vi "Build DashBoard Data.vi"(11 "Dashboard Enables":T2={"Analog Module 1"=[TRUE, TRUE, TRUE, TRUE, TRUE, TRUE, TRUE, TRUE], "Analog Module 2"=[FALSE, FALSE, FALSE, FALSE, FALSE, FALSE, FALSE, FALSE], "Digital Module 1"=TRUE, "Digital Module 2"=FALSE, "Solenoid Module"=TRUE}) -> ()   [LabVIEW 2011]
doc: "This VI builds data and sends it back to the dashboard PC program. By default it sends back the raw values for the first analog, digital, and solenoid module. Modify it to send back the data you want to view. Consider adding higher level data to the Dashboard Datatype.ctl and to this VI. Then update the Dashboard to display the data however you like.\n\nThis software is licensed. Open the labview\\readme\\WPI Robotics Library Open Source License.txt file for more information."
uses:
  DashboardEnable.ctl
  Dashboard Datatype.ctl
  <vilib>/Rock Robotics/WPI/DriverStation/WPI_DriverStationDigitalData.ctl
  System Set Points and States.vi
panel:
  out "Dashboard Data":T1
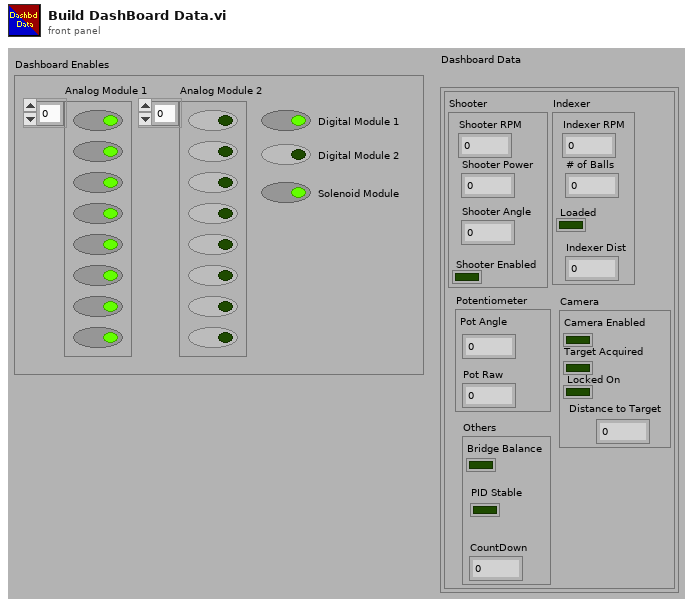
[diagram p1: front panel]
types:
  T1 = typedef "Dashboard Datatype.ctl" = cluster{"Robot Outputs":cluster{"Shooter":cluster{"Shooter RPM":dbl, "Shooter Angle":dbl, "Shooter Power":dbl, "Shooter Enabled":bool}, "Indexer":cluster{"Indexer RPM":dbl, "Loaded":bool, "# of Balls":dbl, "Indexer Dist":dbl}, "Camera":cluster{"Locked On":bool, "Target Acquired":bool, "Camera Enabled":bool, "Distance to Target":dbl}, "Potentiometer":cluster{"Pot Raw":dbl, "Pot Angle":dbl}, "Others":cluster{"CountDown":dbl, "Bridge Balance":bool, "PID Stable":bool}}}
  T2 = typedef "DashboardEnable.ctl" = cluster{"Analog Module 1":bool[], "Analog Module 2":bool[], "Digital Module 1":bool, "Digital Module 2":bool, "Solenoid Module":bool}
  T3 = typedef "WPI_DriverStationDigitalData.ctl" = cluster{"Relay Fwd":u8, "Relay Rev":u8, "GPIO":u16, "GPIO_OE":u16, "PWM":cluster{"PWM[0]":u8, "PWM[1]":u8, "PWM[2]":u8, "PWM[3]":u8, "PWM[4]":u8, "PWM[5]":u8, "PWM[6]":u8, "PWM[7]":u8, "PWM[8]":u8, "PWM[9]":u8}}
  T4 = cluster{"Shooter":cluster{"Shooter RPM":dbl, "Shooter Angle":dbl, "Shooter Power":dbl, "Shooter Enabled":bool}, "Indexer":cluster{"Indexer RPM":dbl, "Loaded":bool, "# of Balls":dbl, "Indexer Dist":dbl}, "Camera":cluster{"Locked On":bool, "Target Acquired":bool, "Camera Enabled":bool, "Distance to Target":dbl}, "Potentiometer":cluster{"Pot Raw":dbl, "Pot Angle":dbl}, "Others":cluster{"CountDown":dbl, "Bridge Balance":bool, "PID Stable":bool}}
  T5 = cluster{"Shooter RPM":dbl, "Shooter Angle":dbl, "Shooter Power":dbl, "Shooter Enabled":bool}
  T6 = cluster{"Indexer RPM":dbl, "Loaded":bool, "# of Balls":dbl, "Indexer Dist":dbl}
  T7 = cluster{"Locked On":bool, "Target Acquired":bool, "Camera Enabled":bool, "Distance to Target":dbl}
  T8 = cluster{"CountDown":dbl, "Bridge Balance":bool, "PID Stable":bool}
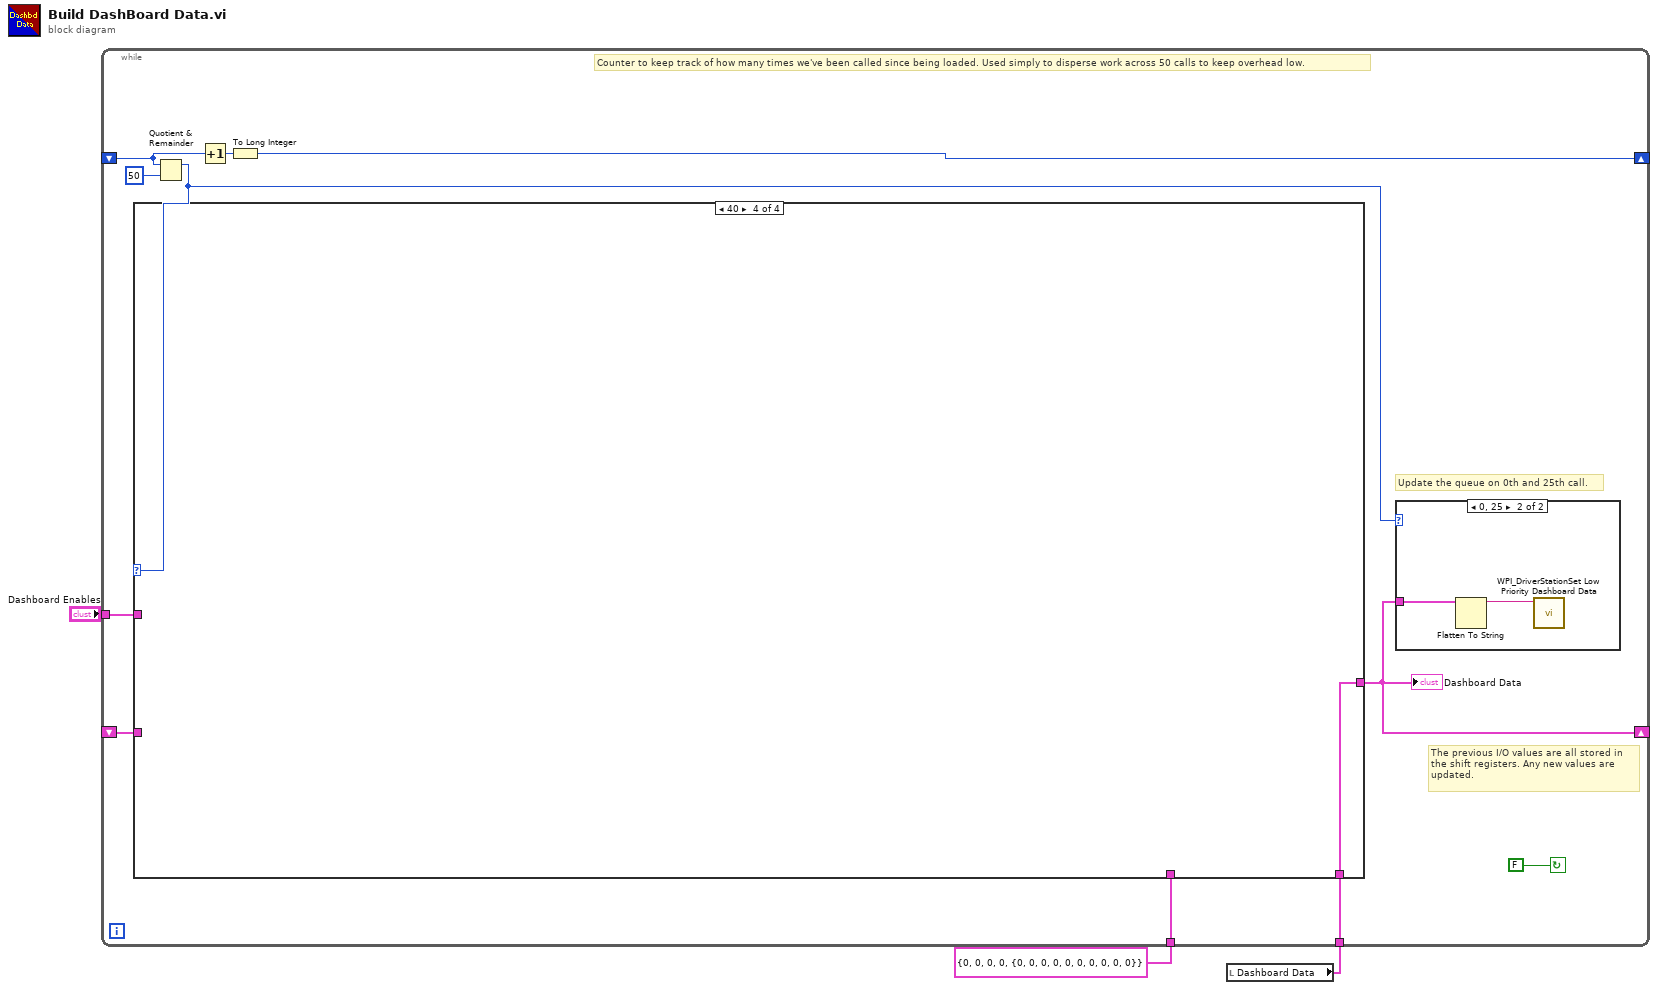
[diagram p0: block diagram]
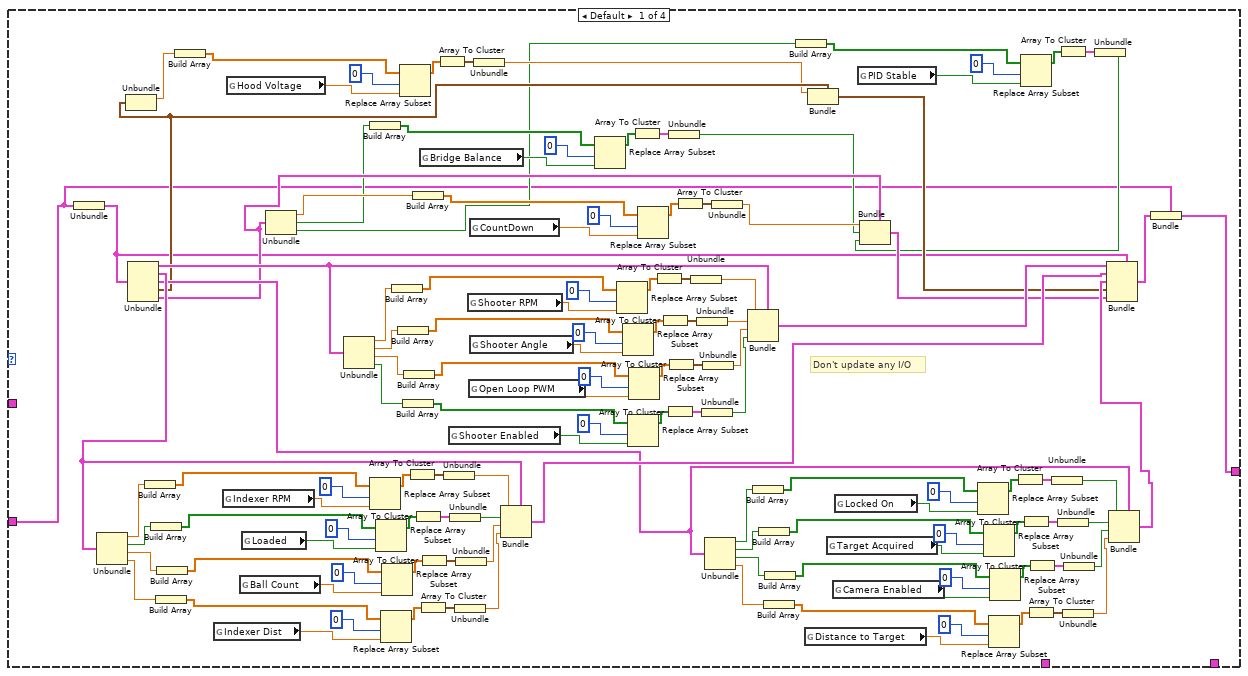
[diagram p3: hidden frame]
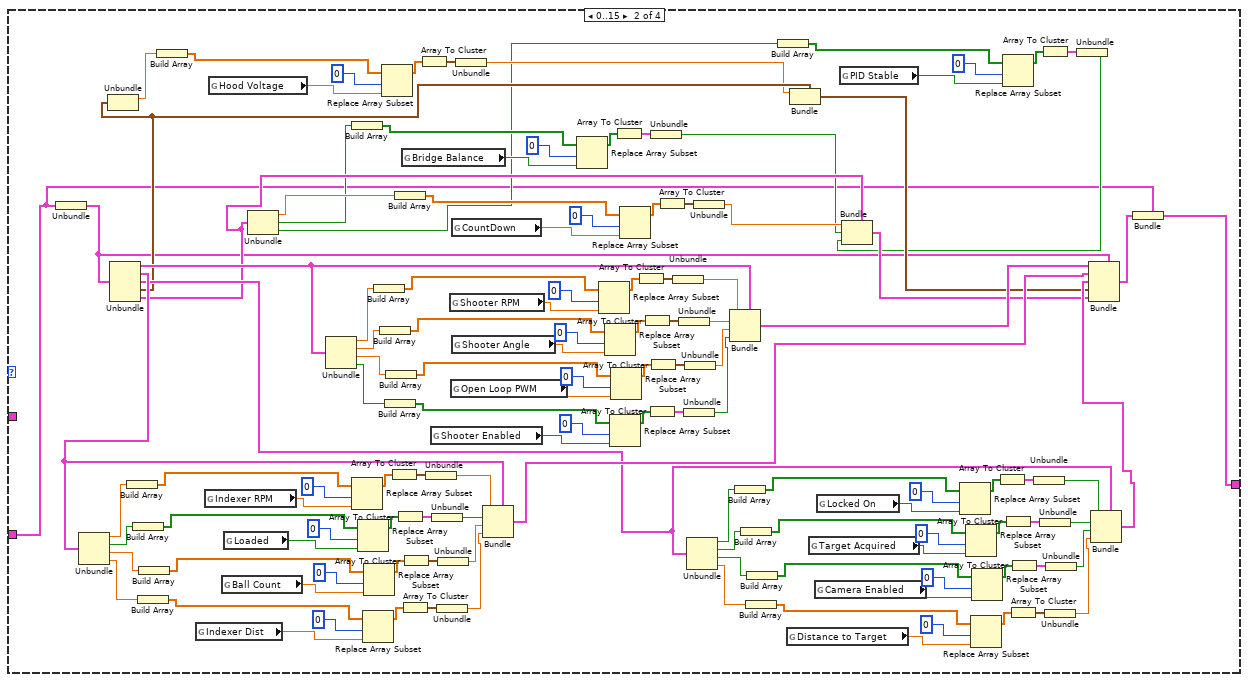
[diagram p4: hidden frame]
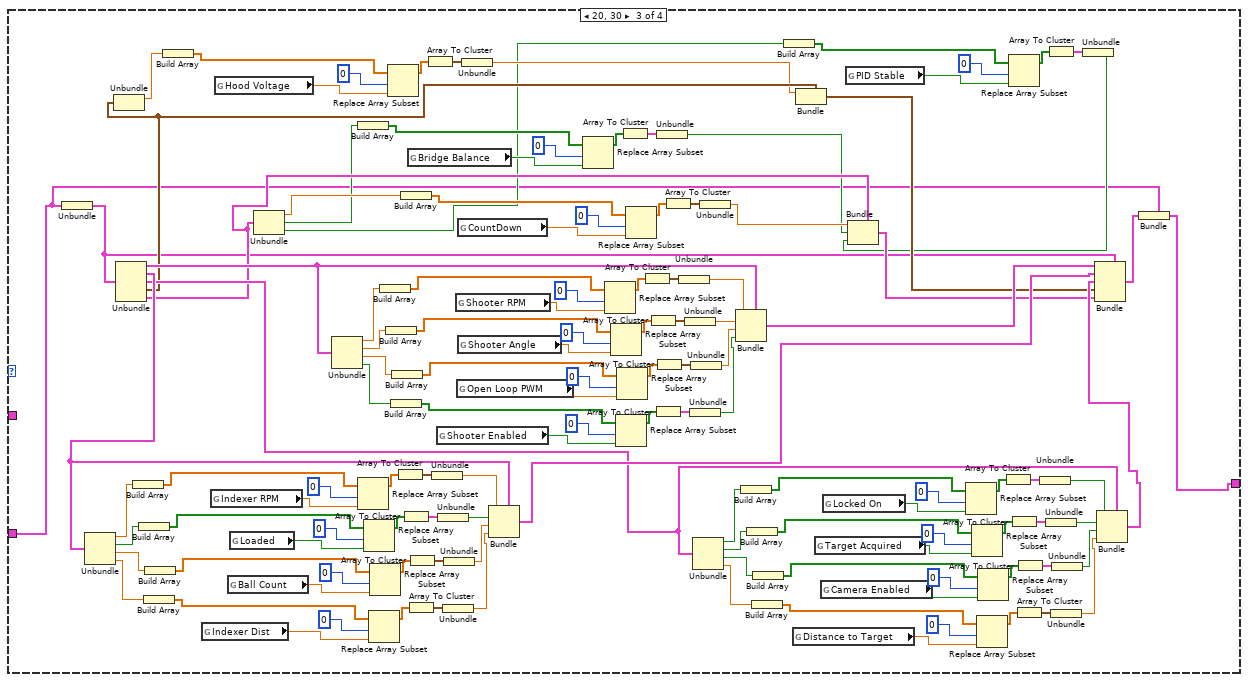
[diagram p5: hidden frame]
diagram:
  n1 = local read "Dashboard Data"() -> (w2:T1)
  n2 = while {
    shift-right: [w7] -> _
    shift-left: _ -> [w9]
    shift-right: [w4] -> _
    shift-left: _ -> [w12]
    tunnel: T3 {"Relay Fwd"=0, "Relay Rev"=0, "GPIO"=0, "GPIO_OE"=0, "PWM"={"PWM[0]"=0, "PWM[1]"=0, "PWM[2]"=0, "PWM[3]"=0, "PWM[4]"=0, "PWM[5]"=0, "PWM[6]"=0, "PWM[7]"=0, "PWM[8]"=0, "PWM[9]"=0}} ("DigitalModule[1]") -> [w11]
    tunnel: w2 -> [w6]
    tunnel: "Dashboard Enables" -> [w5]
    stop <- FALSE continue-if-true
    # "Counter to keep track of how many times we've been called since being loaded. Used simply to disperse work across 50 calls to keep overhead low."
    # "Update the queue on 0th and 25th call."
    # "The previous I/O values are all stored in\nthe shift registers. Any new values are\nupdated."
    n3 = Quotient & Remainder(x=w9, y=50) -> (x-y*floor(x/y)=w8:i32)  [unwired: 1 out]
    n4 = case shown="40" w8 {
      tunnel: [w17 w146 w269 w395] -> w4
      tunnel: w12 -> [w18 w145 w270 _]
      tunnel: w11 -> [_ _ _ _]
      tunnel: w6 -> [_ _ _ w395]
      tunnel: w5 -> [_ _ _ _]
      frame Default {
        # "Don't update any I/O"
        n5 = Unbundle(w18) -> ("Robot Outputs"=w20:T4)
        n6 = Unbundle(w20) -> ("Shooter"=w141:T5, "Indexer"=w84:T6, "Camera"=w54:T7, "Potentiometer"=w31:cluster{"Pot Raw":dbl, "Pot Angle":dbl}, "Others"=w46:T8)
        n7 = Unbundle(w84) -> ("Indexer RPM"=w106:dbl, "Loaded"=w100:bool, "# of Balls"=w92:dbl, "Indexer Dist"=w86:dbl)
        n8 = Unbundle(w31) -> ("Pot Raw"=w32:dbl)  [unwired: 1 out]
        n9 = Build Array(w106) -> (w112:dbl[])
        n10 = Build Array(w100) -> (w105:bool[])
        n11 = Build Array(w86) -> (w91:dbl[])
        n12 = Build Array(w92) -> (w98:dbl[])
        n13 = Build Array(w32) -> (w37:dbl[])
        n14 = global read "System Set Points and States.vi" "Indexer Dist"() -> (w89:dbl)
        n15 = global read "System Set Points and States.vi" "Indexer RPM"() -> (w109:dbl)
        n16 = global read "System Set Points and States.vi" "Hood Voltage"() -> (w35:dbl)
        n17 = global read "System Set Points and States.vi" "Ball Count"() -> (w96:dbl)
        n18 = global read "System Set Points and States.vi" "Loaded"() -> (w103:bool)
        n19 = Unbundle(w46) -> ("CountDown"=w47:dbl, "Bridge Balance"=w39:bool, "PID Stable"=w21:bool)
        n20 = Unbundle(w141) -> ("Shooter RPM"=w134:dbl, "Shooter Angle"=w128:dbl, "Shooter Power"=w120:dbl, "Shooter Enabled"=w114:bool)
        n21 = Build Array(w39) -> (w44:bool[])
        n22 = Replace Array Subset(array=w112, new element=w109, index=0) -> (w107:dbl[])
        n23 = Replace Array Subset(array=w105, new element=w103, index=0) -> (w101:bool[])
        n24 = Replace Array Subset(array=w91, new element=w89, index=0) -> (w87:dbl[])
        n25 = Replace Array Subset(array=w98, new element=w96, index=0) -> (w94:dbl[])
        n26 = Build Array(w134) -> (w142:dbl[])
        n27 = Build Array(w128) -> (w133:dbl[])
        n28 = Replace Array Subset(array=w37, new element=w35, index=0) -> (w33:dbl[])
        n29 = Build Array(w114) -> (w119:bool[])
        n30 = Build Array(w120) -> (w126:dbl[])
        n31 = Array To Cluster(array=w107) -> (cluster=w111:cluster{"[0]":dbl})
        n32 = Build Array(w47) -> (w52:dbl[])
        n33 = Array To Cluster(array=w101) -> (cluster=w104:cluster{"[0]":bool})
        n34 = Array To Cluster(array=w87) -> (cluster=w90:cluster{"[0]":dbl})
        n35 = Array To Cluster(array=w94) -> (cluster=w97:cluster{"[0]":dbl})
        n36 = global read "System Set Points and States.vi" "Bridge Balance"() -> (w42:bool)
        n37 = Array To Cluster(array=w33) -> (cluster=w36:cluster{"[0]":dbl})
        n38 = Unbundle(w111) -> ("[0]"=w110:dbl)
        n39 = global read "System Set Points and States.vi" "Shooter Enabled"() -> (w117:bool)
        n40 = Unbundle(w104) -> ("[0]"=w99:bool)
        n41 = Unbundle(w90) -> ("[0]"=w85:dbl)
        n42 = Unbundle(w97) -> ("[0]"=w93:dbl)
        n43 = global read "System Set Points and States.vi" "Shooter RPM"() -> (w137:dbl)
        n44 = global read "System Set Points and States.vi" "Open Loop PWM"() -> (w124:dbl)
        n45 = global read "System Set Points and States.vi" "CountDown"() -> (w50:dbl)
        n46 = global read "System Set Points and States.vi" "Shooter Angle"() -> (w131:dbl)
        n47 = Unbundle(w36) -> ("[0]"=w30:dbl)
        n48 = Bundle(cluster=w84, "Indexer RPM"=w110, "Loaded"=w99, "# of Balls"=w93, "Indexer Dist"=w85) -> (w83:T6)
        n49 = Replace Array Subset(array=w44, new element=w42, index=0) -> (w40:bool[])
        n50 = Replace Array Subset(array=w142, new element=w137, index=0) -> (w135:dbl[])
        n51 = Replace Array Subset(array=w133, new element=w131, index=0) -> (w129:dbl[])
        n52 = Replace Array Subset(array=w119, new element=w117, index=0) -> (w115:bool[])
        n53 = Replace Array Subset(array=w126, new element=w124, index=0) -> (w122:dbl[])
        n54 = Array To Cluster(array=w40) -> (cluster=w43:cluster{"[0]":bool})
        n55 = Replace Array Subset(array=w52, new element=w50, index=0) -> (w48:dbl[])
        n56 = Array To Cluster(array=w135) -> (cluster=w140:cluster{"[0]":dbl})
        n57 = Array To Cluster(array=w129) -> (cluster=w132:cluster{"[0]":dbl})
        n58 = Array To Cluster(array=w115) -> (cluster=w118:cluster{"[0]":bool})
        n59 = Array To Cluster(array=w122) -> (cluster=w125:cluster{"[0]":dbl})
        n60 = Unbundle(w43) -> ("[0]"=w38:bool)
        n61 = Array To Cluster(array=w48) -> (cluster=w51:cluster{"[0]":dbl})
        n62 = Unbundle(w140) -> ("[0]"=w139:dbl)
        n63 = Unbundle(w132) -> ("[0]"=w127:dbl)
        n64 = Unbundle(w118) -> ("[0]"=w113:bool)
        n65 = Unbundle(w125) -> ("[0]"=w121:dbl)
        n66 = Unbundle(w54) -> ("Locked On"=w76:bool, "Target Acquired"=w70:bool, "Camera Enabled"=w62:bool, "Distance to Target"=w56:dbl)
        n67 = Unbundle(w51) -> ("[0]"=w45:dbl)
        n68 = Bundle(cluster=w141, "Shooter RPM"=w139, "Shooter Angle"=w127, "Shooter Power"=w121, "Shooter Enabled"=w113) -> (w138:T5)
        n69 = Build Array(w76) -> (w82:bool[])
        n70 = Build Array(w70) -> (w75:bool[])
        n71 = Build Array(w56) -> (w61:dbl[])
        n72 = Build Array(w62) -> (w68:bool[])
        n73 = Build Array(w21) -> (w27:bool[])
        n74 = global read "System Set Points and States.vi" "Distance to Target"() -> (w59:dbl)
        n75 = Bundle(cluster=w31, "Pot Raw"=w30) -> (w29:cluster{"Pot Raw":dbl, "Pot Angle":dbl})  [unwired: 1 in]
        n76 = global read "System Set Points and States.vi" "Target Acquired"() -> (w73:bool)
        n77 = global read "System Set Points and States.vi" "Camera Enabled"() -> (w66:bool)
        n78 = global read "System Set Points and States.vi" "Locked On"() -> (w79:bool)
        n79 = global read "System Set Points and States.vi" "PID Stable"() -> (w25:bool)
        n80 = Replace Array Subset(array=w82, new element=w79, index=0) -> (w77:bool[])
        n81 = Replace Array Subset(array=w75, new element=w73, index=0) -> (w71:bool[])
        n82 = Replace Array Subset(array=w61, new element=w59, index=0) -> (w57:dbl[])
        n83 = Replace Array Subset(array=w68, new element=w66, index=0) -> (w64:bool[])
        n84 = Array To Cluster(array=w77) -> (cluster=w81:cluster{"[0]":bool})
        n85 = Replace Array Subset(array=w27, new element=w25, index=0) -> (w23:bool[])
        n86 = Array To Cluster(array=w71) -> (cluster=w74:cluster{"[0]":bool})
        n87 = Array To Cluster(array=w57) -> (cluster=w60:cluster{"[0]":dbl})
        n88 = Array To Cluster(array=w64) -> (cluster=w67:cluster{"[0]":bool})
        n89 = Unbundle(w81) -> ("[0]"=w80:bool)
        n90 = Array To Cluster(array=w23) -> (cluster=w26:cluster{"[0]":bool})
        n91 = Unbundle(w74) -> ("[0]"=w69:bool)
        n92 = Unbundle(w60) -> ("[0]"=w55:dbl)
        n93 = Unbundle(w67) -> ("[0]"=w63:bool)
        n94 = Unbundle(w26) -> ("[0]"=w22:bool)
        n95 = Bundle(cluster=w46, "CountDown"=w45, "Bridge Balance"=w38, "PID Stable"=w22) -> (w28:T8)
        n96 = Bundle(cluster=w54, "Locked On"=w80, "Target Acquired"=w69, "Camera Enabled"=w63, "Distance to Target"=w55) -> (w53:T7)
        n97 = Bundle(cluster=w20, "Shooter"=w138, "Indexer"=w83, "Camera"=w53, "Potentiometer"=w29, "Others"=w28) -> (w19:T4)
        n98 = Bundle(cluster=w18, "Robot Outputs"=w19) -> (w17:T1)
      }
      frame 0..15 {
        n99 = Unbundle(w145) -> ("Robot Outputs"=w144:T4)
        n100 = Unbundle(w144) -> ("Shooter"=w267:T5, "Indexer"=w210:T6, "Camera"=w180:T7, "Potentiometer"=w157:cluster{"Pot Raw":dbl, "Pot Angle":dbl}, "Others"=w172:T8)
        n101 = Unbundle(w210) -> ("Indexer RPM"=w232:dbl, "Loaded"=w226:bool, "# of Balls"=w218:dbl, "Indexer Dist"=w212:dbl)
        n102 = Unbundle(w157) -> ("Pot Raw"=w158:dbl)  [unwired: 1 out]
        n103 = Build Array(w232) -> (w238:dbl[])
        n104 = Build Array(w226) -> (w231:bool[])
        n105 = Build Array(w212) -> (w217:dbl[])
        n106 = Build Array(w218) -> (w224:dbl[])
        n107 = Build Array(w158) -> (w163:dbl[])
        n108 = global read "System Set Points and States.vi" "Indexer Dist"() -> (w215:dbl)
        n109 = global read "System Set Points and States.vi" "Indexer RPM"() -> (w235:dbl)
        n110 = global read "System Set Points and States.vi" "Hood Voltage"() -> (w161:dbl)
        n111 = global read "System Set Points and States.vi" "Ball Count"() -> (w222:dbl)
        n112 = global read "System Set Points and States.vi" "Loaded"() -> (w229:bool)
        n113 = Unbundle(w172) -> ("CountDown"=w173:dbl, "Bridge Balance"=w165:bool, "PID Stable"=w147:bool)
        n114 = Unbundle(w267) -> ("Shooter RPM"=w260:dbl, "Shooter Angle"=w254:dbl, "Shooter Power"=w246:dbl, "Shooter Enabled"=w240:bool)
        n115 = Build Array(w165) -> (w170:bool[])
        n116 = Replace Array Subset(array=w238, new element=w235, index=0) -> (w233:dbl[])
        n117 = Replace Array Subset(array=w231, new element=w229, index=0) -> (w227:bool[])
        n118 = Replace Array Subset(array=w217, new element=w215, index=0) -> (w213:dbl[])
        n119 = Replace Array Subset(array=w224, new element=w222, index=0) -> (w220:dbl[])
        n120 = Build Array(w260) -> (w268:dbl[])
        n121 = Build Array(w254) -> (w259:dbl[])
        n122 = Replace Array Subset(array=w163, new element=w161, index=0) -> (w159:dbl[])
        n123 = Build Array(w240) -> (w245:bool[])
        n124 = Build Array(w246) -> (w252:dbl[])
        n125 = Array To Cluster(array=w233) -> (cluster=w237:cluster{"[0]":dbl})
        n126 = Build Array(w173) -> (w178:dbl[])
        n127 = Array To Cluster(array=w227) -> (cluster=w230:cluster{"[0]":bool})
        n128 = Array To Cluster(array=w213) -> (cluster=w216:cluster{"[0]":dbl})
        n129 = Array To Cluster(array=w220) -> (cluster=w223:cluster{"[0]":dbl})
        n130 = global read "System Set Points and States.vi" "Bridge Balance"() -> (w168:bool)
        n131 = Array To Cluster(array=w159) -> (cluster=w162:cluster{"[0]":dbl})
        n132 = Unbundle(w237) -> ("[0]"=w236:dbl)
        n133 = global read "System Set Points and States.vi" "Shooter Enabled"() -> (w243:bool)
        n134 = Unbundle(w230) -> ("[0]"=w225:bool)
        n135 = Unbundle(w216) -> ("[0]"=w211:dbl)
        n136 = Unbundle(w223) -> ("[0]"=w219:dbl)
        n137 = global read "System Set Points and States.vi" "Shooter RPM"() -> (w263:dbl)
        n138 = global read "System Set Points and States.vi" "Open Loop PWM"() -> (w250:dbl)
        n139 = global read "System Set Points and States.vi" "CountDown"() -> (w176:dbl)
        n140 = global read "System Set Points and States.vi" "Shooter Angle"() -> (w257:dbl)
        n141 = Unbundle(w162) -> ("[0]"=w156:dbl)
        n142 = Bundle(cluster=w210, "Indexer RPM"=w236, "Loaded"=w225, "# of Balls"=w219, "Indexer Dist"=w211) -> (w209:T6)
        n143 = Replace Array Subset(array=w170, new element=w168, index=0) -> (w166:bool[])
        n144 = Replace Array Subset(array=w268, new element=w263, index=0) -> (w261:dbl[])
        n145 = Replace Array Subset(array=w259, new element=w257, index=0) -> (w255:dbl[])
        n146 = Replace Array Subset(array=w245, new element=w243, index=0) -> (w241:bool[])
        n147 = Replace Array Subset(array=w252, new element=w250, index=0) -> (w248:dbl[])
        n148 = Array To Cluster(array=w166) -> (cluster=w169:cluster{"[0]":bool})
        n149 = Replace Array Subset(array=w178, new element=w176, index=0) -> (w174:dbl[])
        n150 = Array To Cluster(array=w261) -> (cluster=w266:cluster{"[0]":dbl})
        n151 = Array To Cluster(array=w255) -> (cluster=w258:cluster{"[0]":dbl})
        n152 = Array To Cluster(array=w241) -> (cluster=w244:cluster{"[0]":bool})
        n153 = Array To Cluster(array=w248) -> (cluster=w251:cluster{"[0]":dbl})
        n154 = Unbundle(w169) -> ("[0]"=w164:bool)
        n155 = Array To Cluster(array=w174) -> (cluster=w177:cluster{"[0]":dbl})
        n156 = Unbundle(w266) -> ("[0]"=w265:dbl)
        n157 = Unbundle(w258) -> ("[0]"=w253:dbl)
        n158 = Unbundle(w244) -> ("[0]"=w239:bool)
        n159 = Unbundle(w251) -> ("[0]"=w247:dbl)
        n160 = Unbundle(w180) -> ("Locked On"=w202:bool, "Target Acquired"=w196:bool, "Camera Enabled"=w188:bool, "Distance to Target"=w182:dbl)
        n161 = Unbundle(w177) -> ("[0]"=w171:dbl)
        n162 = Bundle(cluster=w267, "Shooter RPM"=w265, "Shooter Angle"=w253, "Shooter Power"=w247, "Shooter Enabled"=w239) -> (w264:T5)
        n163 = Build Array(w202) -> (w208:bool[])
        n164 = Build Array(w196) -> (w201:bool[])
        n165 = Build Array(w182) -> (w187:dbl[])
        n166 = Build Array(w188) -> (w194:bool[])
        n167 = Build Array(w147) -> (w153:bool[])
        n168 = global read "System Set Points and States.vi" "Distance to Target"() -> (w185:dbl)
        n169 = Bundle(cluster=w157, "Pot Raw"=w156) -> (w155:cluster{"Pot Raw":dbl, "Pot Angle":dbl})  [unwired: 1 in]
        n170 = global read "System Set Points and States.vi" "Target Acquired"() -> (w199:bool)
        n171 = global read "System Set Points and States.vi" "Camera Enabled"() -> (w192:bool)
        n172 = global read "System Set Points and States.vi" "Locked On"() -> (w205:bool)
        n173 = global read "System Set Points and States.vi" "PID Stable"() -> (w151:bool)
        n174 = Replace Array Subset(array=w208, new element=w205, index=0) -> (w203:bool[])
        n175 = Replace Array Subset(array=w201, new element=w199, index=0) -> (w197:bool[])
        n176 = Replace Array Subset(array=w187, new element=w185, index=0) -> (w183:dbl[])
        n177 = Replace Array Subset(array=w194, new element=w192, index=0) -> (w190:bool[])
        n178 = Array To Cluster(array=w203) -> (cluster=w207:cluster{"[0]":bool})
        n179 = Replace Array Subset(array=w153, new element=w151, index=0) -> (w149:bool[])
        n180 = Array To Cluster(array=w197) -> (cluster=w200:cluster{"[0]":bool})
        n181 = Array To Cluster(array=w183) -> (cluster=w186:cluster{"[0]":dbl})
        n182 = Array To Cluster(array=w190) -> (cluster=w193:cluster{"[0]":bool})
        n183 = Unbundle(w207) -> ("[0]"=w206:bool)
        n184 = Array To Cluster(array=w149) -> (cluster=w152:cluster{"[0]":bool})
        n185 = Unbundle(w200) -> ("[0]"=w195:bool)
        n186 = Unbundle(w186) -> ("[0]"=w181:dbl)
        n187 = Unbundle(w193) -> ("[0]"=w189:bool)
        n188 = Unbundle(w152) -> ("[0]"=w148:bool)
        n189 = Bundle(cluster=w172, "CountDown"=w171, "Bridge Balance"=w164, "PID Stable"=w148) -> (w154:T8)
        n190 = Bundle(cluster=w180, "Locked On"=w206, "Target Acquired"=w195, "Camera Enabled"=w189, "Distance to Target"=w181) -> (w179:T7)
        n191 = Bundle(cluster=w144, "Shooter"=w264, "Indexer"=w209, "Camera"=w179, "Potentiometer"=w155, "Others"=w154) -> (w143:T4)
        n192 = Bundle(cluster=w145, "Robot Outputs"=w143) -> (w146:T1)
      }
      frame 20, 30 {
        n193 = Unbundle(w270) -> ("Robot Outputs"=w272:T4)
        n194 = Unbundle(w272) -> ("Shooter"=w393:T5, "Indexer"=w336:T6, "Camera"=w306:T7, "Potentiometer"=w283:cluster{"Pot Raw":dbl, "Pot Angle":dbl}, "Others"=w298:T8)
        n195 = Unbundle(w336) -> ("Indexer RPM"=w358:dbl, "Loaded"=w352:bool, "# of Balls"=w344:dbl, "Indexer Dist"=w338:dbl)
        n196 = Unbundle(w283) -> ("Pot Raw"=w284:dbl)  [unwired: 1 out]
        n197 = Build Array(w358) -> (w364:dbl[])
        n198 = Build Array(w352) -> (w357:bool[])
        n199 = Build Array(w338) -> (w343:dbl[])
        n200 = Build Array(w344) -> (w350:dbl[])
        n201 = Build Array(w284) -> (w289:dbl[])
        n202 = global read "System Set Points and States.vi" "Indexer Dist"() -> (w341:dbl)
        n203 = global read "System Set Points and States.vi" "Indexer RPM"() -> (w361:dbl)
        n204 = global read "System Set Points and States.vi" "Hood Voltage"() -> (w287:dbl)
        n205 = global read "System Set Points and States.vi" "Ball Count"() -> (w348:dbl)
        n206 = global read "System Set Points and States.vi" "Loaded"() -> (w355:bool)
        n207 = Unbundle(w298) -> ("CountDown"=w299:dbl, "Bridge Balance"=w291:bool, "PID Stable"=w273:bool)
        n208 = Unbundle(w393) -> ("Shooter RPM"=w386:dbl, "Shooter Angle"=w380:dbl, "Shooter Power"=w372:dbl, "Shooter Enabled"=w366:bool)
        n209 = Build Array(w291) -> (w296:bool[])
        n210 = Replace Array Subset(array=w364, new element=w361, index=0) -> (w359:dbl[])
        n211 = Replace Array Subset(array=w357, new element=w355, index=0) -> (w353:bool[])
        n212 = Replace Array Subset(array=w343, new element=w341, index=0) -> (w339:dbl[])
        n213 = Replace Array Subset(array=w350, new element=w348, index=0) -> (w346:dbl[])
        n214 = Build Array(w386) -> (w394:dbl[])
        n215 = Build Array(w380) -> (w385:dbl[])
        n216 = Replace Array Subset(array=w289, new element=w287, index=0) -> (w285:dbl[])
        n217 = Build Array(w366) -> (w371:bool[])
        n218 = Build Array(w372) -> (w378:dbl[])
        n219 = Array To Cluster(array=w359) -> (cluster=w363:cluster{"[0]":dbl})
        n220 = Build Array(w299) -> (w304:dbl[])
        n221 = Array To Cluster(array=w353) -> (cluster=w356:cluster{"[0]":bool})
        n222 = Array To Cluster(array=w339) -> (cluster=w342:cluster{"[0]":dbl})
        n223 = Array To Cluster(array=w346) -> (cluster=w349:cluster{"[0]":dbl})
        n224 = global read "System Set Points and States.vi" "Bridge Balance"() -> (w294:bool)
        n225 = Array To Cluster(array=w285) -> (cluster=w288:cluster{"[0]":dbl})
        n226 = Unbundle(w363) -> ("[0]"=w362:dbl)
        n227 = global read "System Set Points and States.vi" "Shooter Enabled"() -> (w369:bool)
        n228 = Unbundle(w356) -> ("[0]"=w351:bool)
        n229 = Unbundle(w342) -> ("[0]"=w337:dbl)
        n230 = Unbundle(w349) -> ("[0]"=w345:dbl)
        n231 = global read "System Set Points and States.vi" "Shooter RPM"() -> (w389:dbl)
        n232 = global read "System Set Points and States.vi" "Open Loop PWM"() -> (w376:dbl)
        n233 = global read "System Set Points and States.vi" "CountDown"() -> (w302:dbl)
        n234 = global read "System Set Points and States.vi" "Shooter Angle"() -> (w383:dbl)
        n235 = Unbundle(w288) -> ("[0]"=w282:dbl)
        n236 = Bundle(cluster=w336, "Indexer RPM"=w362, "Loaded"=w351, "# of Balls"=w345, "Indexer Dist"=w337) -> (w335:T6)
        n237 = Replace Array Subset(array=w296, new element=w294, index=0) -> (w292:bool[])
        n238 = Replace Array Subset(array=w394, new element=w389, index=0) -> (w387:dbl[])
        n239 = Replace Array Subset(array=w385, new element=w383, index=0) -> (w381:dbl[])
        n240 = Replace Array Subset(array=w371, new element=w369, index=0) -> (w367:bool[])
        n241 = Replace Array Subset(array=w378, new element=w376, index=0) -> (w374:dbl[])
        n242 = Array To Cluster(array=w292) -> (cluster=w295:cluster{"[0]":bool})
        n243 = Replace Array Subset(array=w304, new element=w302, index=0) -> (w300:dbl[])
        n244 = Array To Cluster(array=w387) -> (cluster=w392:cluster{"[0]":dbl})
        n245 = Array To Cluster(array=w381) -> (cluster=w384:cluster{"[0]":dbl})
        n246 = Array To Cluster(array=w367) -> (cluster=w370:cluster{"[0]":bool})
        n247 = Array To Cluster(array=w374) -> (cluster=w377:cluster{"[0]":dbl})
        n248 = Unbundle(w295) -> ("[0]"=w290:bool)
        n249 = Array To Cluster(array=w300) -> (cluster=w303:cluster{"[0]":dbl})
        n250 = Unbundle(w392) -> ("[0]"=w391:dbl)
        n251 = Unbundle(w384) -> ("[0]"=w379:dbl)
        n252 = Unbundle(w370) -> ("[0]"=w365:bool)
        n253 = Unbundle(w377) -> ("[0]"=w373:dbl)
        n254 = Unbundle(w306) -> ("Locked On"=w328:bool, "Target Acquired"=w322:bool, "Camera Enabled"=w314:bool, "Distance to Target"=w308:dbl)
        n255 = Unbundle(w303) -> ("[0]"=w297:dbl)
        n256 = Bundle(cluster=w393, "Shooter RPM"=w391, "Shooter Angle"=w379, "Shooter Power"=w373, "Shooter Enabled"=w365) -> (w390:T5)
        n257 = Build Array(w328) -> (w334:bool[])
        n258 = Build Array(w322) -> (w327:bool[])
        n259 = Build Array(w308) -> (w313:dbl[])
        n260 = Build Array(w314) -> (w320:bool[])
        n261 = Build Array(w273) -> (w279:bool[])
        n262 = global read "System Set Points and States.vi" "Distance to Target"() -> (w311:dbl)
        n263 = Bundle(cluster=w283, "Pot Raw"=w282) -> (w281:cluster{"Pot Raw":dbl, "Pot Angle":dbl})  [unwired: 1 in]
        n264 = global read "System Set Points and States.vi" "Target Acquired"() -> (w325:bool)
        n265 = global read "System Set Points and States.vi" "Camera Enabled"() -> (w318:bool)
        n266 = global read "System Set Points and States.vi" "Locked On"() -> (w331:bool)
        n267 = global read "System Set Points and States.vi" "PID Stable"() -> (w277:bool)
        n268 = Replace Array Subset(array=w334, new element=w331, index=0) -> (w329:bool[])
        n269 = Replace Array Subset(array=w327, new element=w325, index=0) -> (w323:bool[])
        n270 = Replace Array Subset(array=w313, new element=w311, index=0) -> (w309:dbl[])
        n271 = Replace Array Subset(array=w320, new element=w318, index=0) -> (w316:bool[])
        n272 = Array To Cluster(array=w329) -> (cluster=w333:cluster{"[0]":bool})
        n273 = Replace Array Subset(array=w279, new element=w277, index=0) -> (w275:bool[])
        n274 = Array To Cluster(array=w323) -> (cluster=w326:cluster{"[0]":bool})
        n275 = Array To Cluster(array=w309) -> (cluster=w312:cluster{"[0]":dbl})
        n276 = Array To Cluster(array=w316) -> (cluster=w319:cluster{"[0]":bool})
        n277 = Unbundle(w333) -> ("[0]"=w332:bool)
        n278 = Array To Cluster(array=w275) -> (cluster=w278:cluster{"[0]":bool})
        n279 = Unbundle(w326) -> ("[0]"=w321:bool)
        n280 = Unbundle(w312) -> ("[0]"=w307:dbl)
        n281 = Unbundle(w319) -> ("[0]"=w315:bool)
        n282 = Unbundle(w278) -> ("[0]"=w274:bool)
        n283 = Bundle(cluster=w298, "CountDown"=w297, "Bridge Balance"=w290, "PID Stable"=w274) -> (w280:T8)
        n284 = Bundle(cluster=w306, "Locked On"=w332, "Target Acquired"=w321, "Camera Enabled"=w315, "Distance to Target"=w307) -> (w305:T7)
        n285 = Bundle(cluster=w272, "Shooter"=w390, "Indexer"=w335, "Camera"=w305, "Potentiometer"=w281, "Others"=w280) -> (w271:T4)
        n286 = Bundle(cluster=w270, "Robot Outputs"=w271) -> (w269:T1)
      }
      frame 40 {
      }
    }
    "Dashboard Data" <- w4
    n287 = Increment(x=w9) -> (x+1=w14:i32)
    n288 = To Long Integer(number=w14) -> (32bit integer=w7:i32)
    n289 = case shown="0, 25" w8 {
      tunnel: w4 -> [_ w16]
      frame Default {
      }
      frame 0, 25 {
        n290 = Flatten To String(anything=w16) -> (data string=w15:string)  [unwired: 1 in, 4 out]
        n291 = call <vilib>:"WPI_DriverStationSet Low Priority Dashboard Data.vi"("User Data"=w15) -> ()  [unwired: 1 in, 10 out]
      }
    }
  }
